vi "OpenCV PyrDown.vi"(8 "error in (no error)":errorcluster, 10 "Image Dst":T1, 11 "Image Src":T1) -> (0 "error out":errorcluster, 3 "Image Dst Out":T1)   [LabVIEW 2023]
uses:
  <vilib>/vision/Image Controls.llb/IMAQ Image.ctl
  WrapperDLL/x64/Release/Wrapper.dll
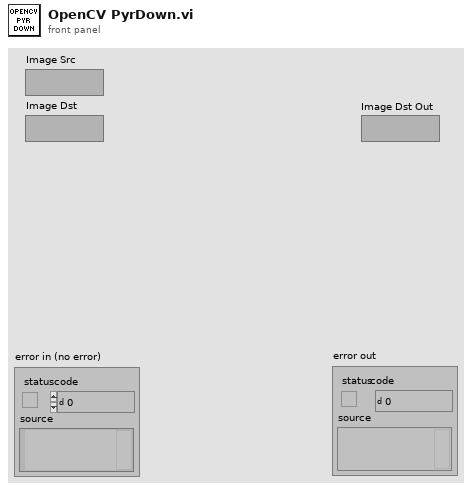
[diagram p1: front panel]
types:
  T1 = typedef "IMAQ Image.ctl" = refnum<image>
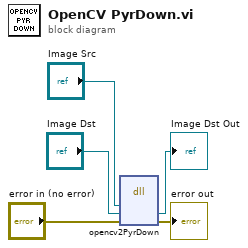
[diagram p0: block diagram]
diagram:
  n1 = dll-call lib="C:/Users/Andrey/Desktop/xe2/WrapperDLL/x64/Release/Wrapper.dll" fn="opencv2PyrDown"("src"="Image Src", "dst"="Image Dst", "error"="error in (no error)") -> ("dst"=→"Image Dst Out":T1, "error"=→"error out":errorcluster)  [unwired: 5 in, 2 out]
